vi "Get VI Event Structure Reference.vi"(8 "error in (no error)":errorcluster, 11 "JKI SM in":refnum<class "JKI SM.lvclass">) -> (0 "error out":errorcluster, 2 "Event Structure ref":refnum<vi>, 3 "JKI SM out":refnum<class "JKI SM.lvclass">)   [LabVIEW 2020, in "JKI State Machine API.lvlib" / "JKI SM.lvclass"]
uses:
  JKI SM.lvclass
  JKI SM.lvclass/JKI SM.ctl
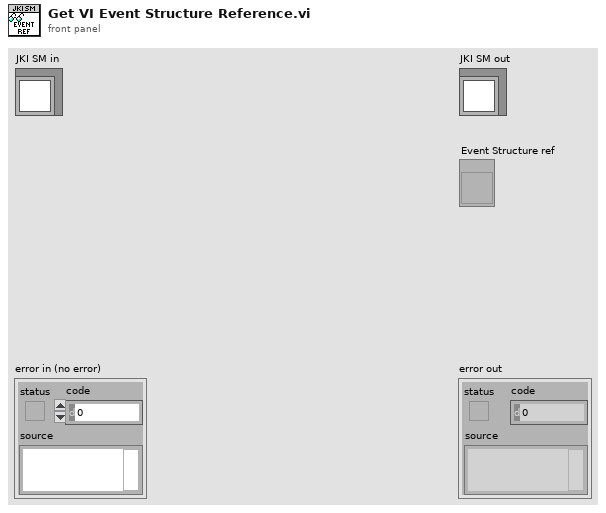
[diagram p1: front panel]
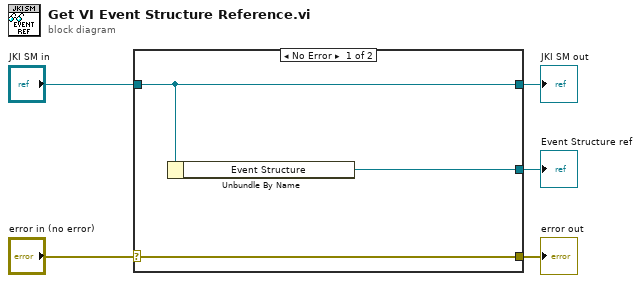
[diagram p0: block diagram]
diagram:
  n1 = case shown="No Error" "error in (no error)" {
    selector: "error in (no error)" -> [w8 w9]
    tunnel: [w8 w9] -> w4
    tunnel: [w7 w10] -> w2
    tunnel: "JKI SM in" -> [w7 w10]
    tunnel: [w6 _] -> w1
    frame No Error {
      n2 = Unbundle By Name(w7) -> ("Event Structure"=w6:refnum<vi>)
    }
    frame Error {
    }
  }
  "error out" <- w4
  "JKI SM out" <- w2
  "Event Structure ref" <- w1
